vi "dfd_Multirate Filter to Nyquist.vi"(7 "#band":i32=2, 8 "error in (no error)":errorcluster, 11 "h in":dbl[](array[numeric])) -> (0 "error out":errorcluster, 3 "h out":dbl[](array[numeric]))   [LabVIEW 2017, in "NI_DigFilter_Process.lvlib"]
uses:
  <vilib>/addons/Digital Filter Design/NI_DigFilter_Process.lvlib
  <vilib>/Analysis/2dsp.llb/Inverse Real FFT.vi
  <vilib>/addons/Digital Filter Design/NI_DigFilterLicensed.lvlib
  <vilib>/Analysis/NI_AALPro.lvlib
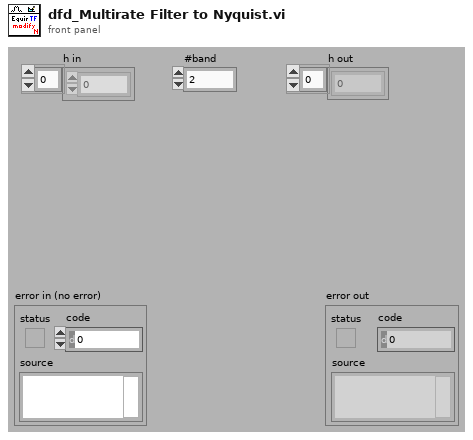
[diagram p1: front panel]
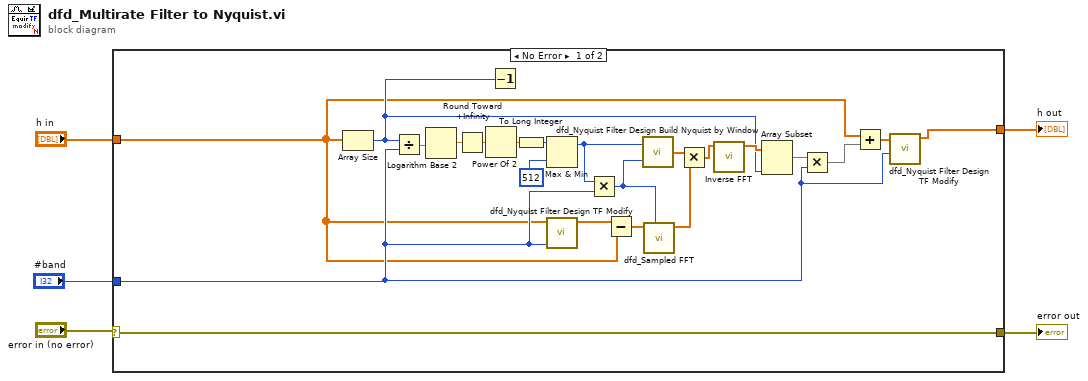
[diagram p0: block diagram]
diagram:
  n1 = case shown="No Error" "error in (no error)" {
    selector: "error in (no error)" -> [w7 w28]
    tunnel: "#band" -> [w9 _]
    tunnel: "h in" -> [w6 _]
    tunnel: [w7 w28] -> w3
    tunnel: [w8 _] -> w2
    frame No Error {
      n2 = Array Size(array=w6) -> (size(s)=w14:i32)
      n3 = Divide(x=w14, y=w9) -> (x/y=w26:dbl)
      n4 = Logarithm Base 2(1:w26) -> (0:w25:dbl)
      n5 = Round Toward +Infinity(x=w25) -> (ceil(x): smallest int >= x=w24:dbl)
      n6 = Power Of 2(x=w24) -> (2^x=w23:dbl)
      n7 = Decrement(x=w14) -> ()  [unwired: 1 out]
      n8 = To Long Integer(number=w23) -> (32bit integer=w20:i32)
      n9 = Max & Min(x=w20, y=512 ("# freq bins (512)")) -> (max(x,y)=w13:i32)  [unwired: 1 out]
      n10 = call <vilib>:"dfd_Nyquist Filter Design TF Modify.vi"("band"=w9, "tf"=w6) -> ("new tf"=w17:dbl[])  [unwired: 1 in, 8 out]
      n11 = Multiply(x=w13, y=w9) -> (x*y=w10:i32)
      n12 = Subtract(x=w17, y=w6) -> (x-y=w18:dbl[])
      n13 = call <vilib>:"dfd_Nyquist Filter Design Build Nyquist by Window.vi"("FFT size"=w10, "window length"=w13) -> ("nyquist filter spectrum"=w16:dbl[])
      n14 = call <vilib>:"dfd_Sampled FFT.vi"("# freq bins (512)"=w10, "h[n]"=w18) -> ("FFT {X}"=w12:cdb[])  [unwired: 2 in, 7 out]
      n15 = Multiply(x=w16, y=w12) -> (x*y=w15:cdb[])
      n16 = call-poly <vilib>:"Inverse FFT.vi"("FFT {X}"=w15) -> ("X"=w27:dbl[])  [unwired: 1 in, 9 out]
      n17 = Array Subset(array=w27, length=w14) -> (w22:dbl[])  [unwired: 1 in]
      n18 = Multiply(x=w22, y=w9) -> (x*y=w11:dbl[])
      n19 = Add(x=w6, y=w11) -> (x+y=w21:dbl[])
      n20 = call <vilib>:"dfd_Nyquist Filter Design TF Modify.vi"("band"=w9, "tf"=w21) -> ("new tf"=w8:dbl[])  [unwired: 1 in, 8 out]
    }
    frame Error {
    }
  }
  "error out" <- w3
  "h out" <- w2
